vi "combinatie.vi"() -> ()   [LabVIEW 2019]
panel:
  in  "linksachter":bool
  in  "rechtsachter":bool
  in  "rechtsvooruit":bool
  in  "linksvooruit":bool
  in  "rechts":bool
  in  "links":bool
  out "port":u16
  in  "stop 2":bool
  out "data out":string
  in  "achteruit":bool
  in  "vooruit":bool
  in  "stop":bool
  # "sender"
  # "receiver"
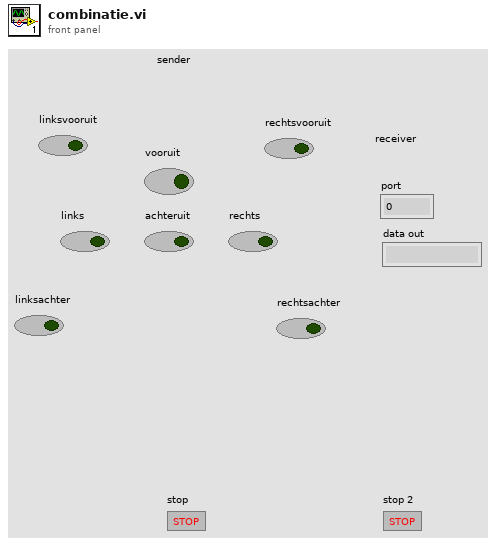
[diagram p1: front panel]
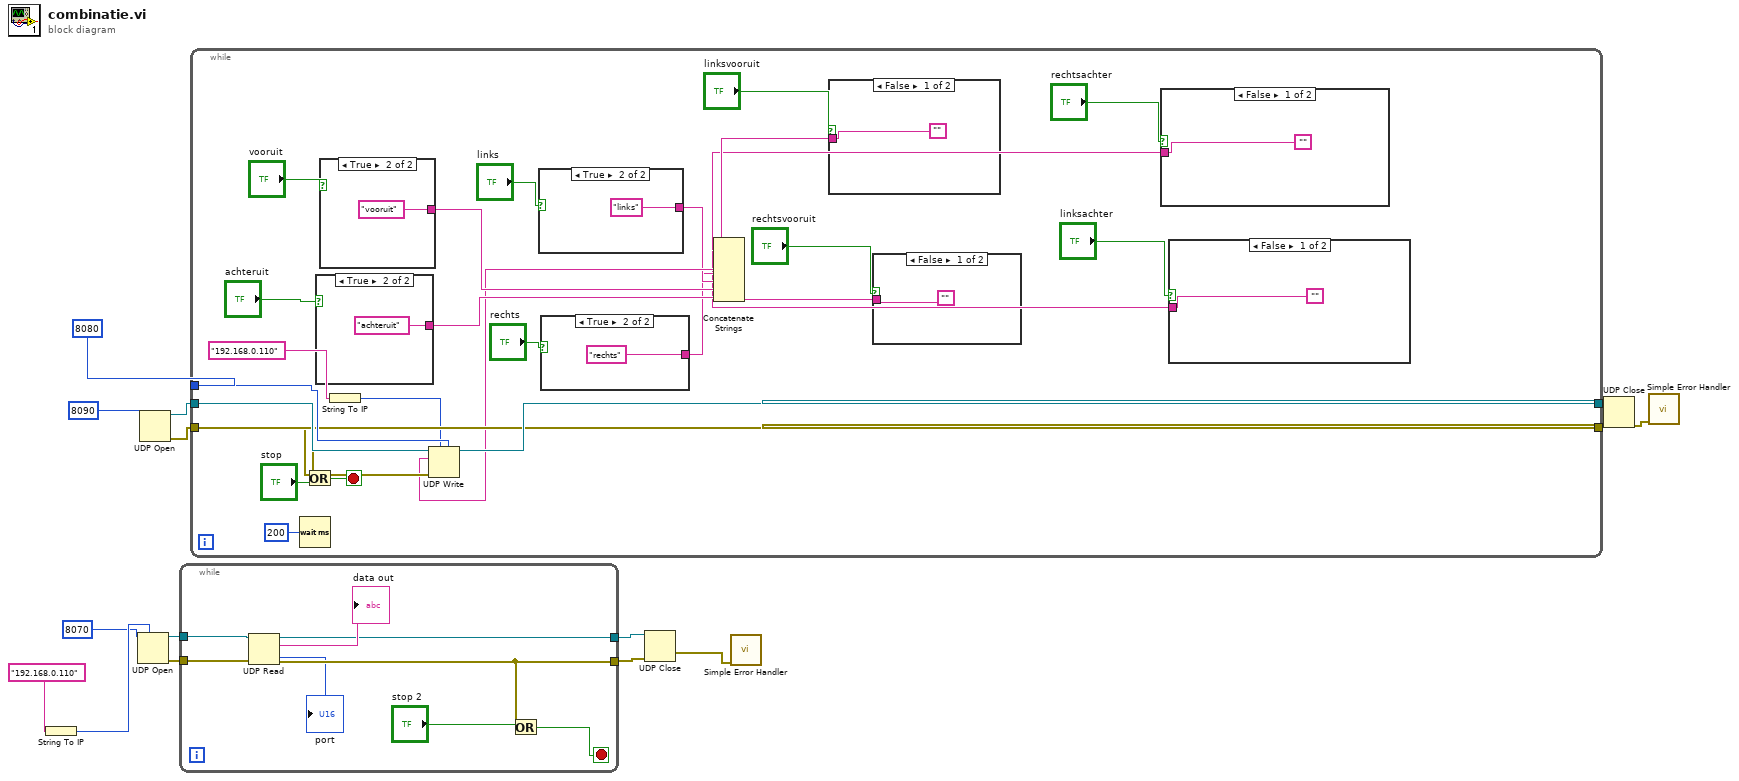
[diagram p0: block diagram]
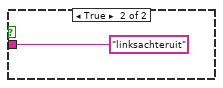
[diagram p2: hidden frame]
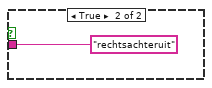
[diagram p3: hidden frame]
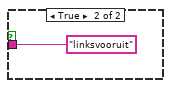
[diagram p4: hidden frame]
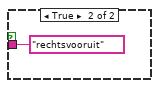
[diagram p5: hidden frame]
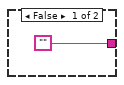
[diagram p6: hidden frame]
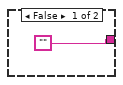
[diagram p7: hidden frame]
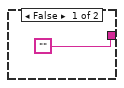
[diagram p8: hidden frame]
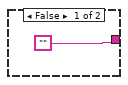
[diagram p9: hidden frame]
diagram:
  n1 = String To IP(1:"192.168.0.110") -> (0:w5:u32)
  n2 = UDP Open(7:w5, 11:u16 8070 ("port")) -> (port=w3:refnum<k16>, 0:w2:errorcluster)  [unwired: 3 in, 1 out]
  n3 = UDP Open(11:8090) -> (port=w14:refnum<k16>, 0:w13:errorcluster)  [unwired: 4 in, 1 out]
  n4 = while {
    tunnel: [w20] -> w8
    tunnel: [w19] -> w7
    tunnel: w3 -> [w18]
    tunnel: w2 -> [w17]
    stop <- w21 stop-if-true
    n5 = UDP Read(connection ID=w18, 8:w17) -> (data out=→"data out":string, error out=w20:errorcluster, 3:w19:refnum<k16>, 4:→"port":u16)  [unwired: 2 in, 1 out]
    n6 = Or(x=w20, y="stop 2") -> (x .or. y?=w21:bool)
  }
  n7 = while {
    tunnel: w14 -> [w50]
    tunnel: w13 -> [w49]
    tunnel: 8080 -> [w45]
    tunnel: [w44] -> w11
    tunnel: [w43] -> w10
    stop <- w47 stop-if-true
    n8 = Wait (ms)(milliseconds to wait=200) -> ()  [unwired: 1 out]
    n9 = case shown="True" "achteruit" {
      tunnel: ["" "achteruit"] -> w39
      frame False {
      }
      frame True {
      }
    }
    n10 = case shown="True" "vooruit" {
      tunnel: ["" "vooruit"] -> w40
      frame False {
      }
      frame True {
      }
    }
    n11 = String To IP(1:"192.168.0.110") -> (0:w36:u32)
    n12 = case shown="True" "links" {
      tunnel: ["" "links"] -> w35
      frame False {
      }
      frame True {
      }
    }
    n13 = case shown="True" "rechts" {
      tunnel: ["" "rechts"] -> w33
      frame False {
      }
      frame True {
      }
    }
    n14 = case shown="False" "linksvooruit" {
      tunnel: ["" "linksvooruit"] -> w29
      frame False {
      }
      frame True {
      }
    }
    n15 = case shown="False" "rechtsvooruit" {
      tunnel: ["" "rechtsvooruit"] -> w30
      frame False {
      }
      frame True {
      }
    }
    n16 = case shown="False" "rechtsachter" {
      tunnel: ["" "rechtsachteruit"] -> w27
      frame False {
      }
      frame True {
      }
    }
    n17 = case shown="False" "linksachter" {
      tunnel: ["" "linksachteruit"] -> w26
      frame False {
      }
      frame True {
      }
    }
    n18 = Concatenate Strings(w26, w27, w29, w30, w33, w35, w40, w39) -> (w38:string)
    n19 = UDP Write(address=w36, port or service name=w45, connection ID=w50, data in=w38, 8:w49) -> (error out=w43:errorcluster, 3:w44:refnum<k16>)  [unwired: 1 in]
    n20 = Or(x=w43, y="stop") -> (x .or. y?=w47:bool)
  }
  n21 = UDP Close(connection ID=w7, 8:w8) -> (error out=w1:errorcluster)  [unwired: 1 out]
  n22 = call <vilib>:"Simple Error Handler.vi"("error in (no error)"=w1) -> ()  [unwired: 4 in, 5 out]
  n23 = UDP Close(connection ID=w11, 8:w10) -> (error out=w9:errorcluster)  [unwired: 1 out]
  n24 = call <vilib>:"Simple Error Handler.vi"("error in (no error)"=w9) -> ()  [unwired: 4 in, 5 out]
